vi "Measurement Parser.vi"(8 "error in (no error)":errorcluster, 9 "Universal Power Meter.lvlib:Universal Card.lvclass":refnum<class "Universal Card.lvclass">, 10 "Data Array":dbl[](array[numeric]), 11 "Yokogawa WT500 in":refnum<class "Yokogawa WT500.lvclass">) -> (0 "error out":errorcluster, 2 "Waveform Graph":dynamicdata(graph), 3 "Yokogawa WT500 out":refnum<class "Yokogawa WT500.lvclass">)   [LabVIEW 2013, in "Universal Power Meter.lvlib" / "Yokogawa WT500.lvlib" / "Yokogawa WT500.lvclass"]
uses:
  Yokogawa WT500.lvclass
  Universal Card Class/Universal Card.lvclass
  Measured Value Header Control.ctl
  Universal Card Class/Universal Card.lvclass/Universal Card.ctl
  Generic Instrument/Generic Card/Generic Card.lvclass/Generic Card.ctl
  Generic Instrument/Generic Card/Generic Card.lvclass
  Data Logger/Data Logger.lvclass
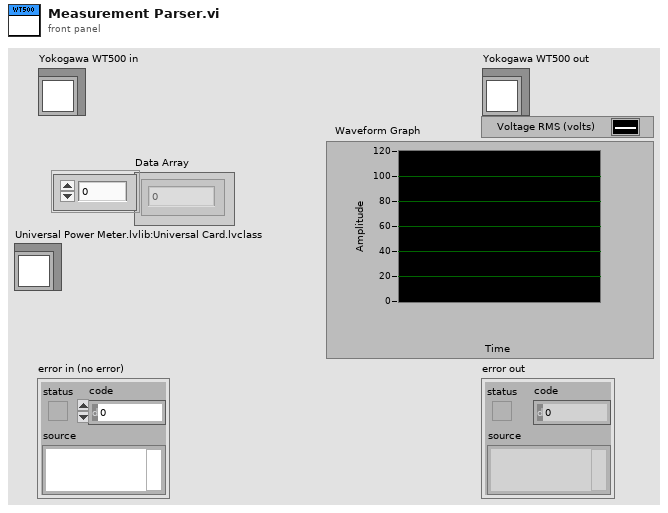
[diagram p1: front panel]
types:
  T1 = typedef "Measured Value Header Control.ctl" = enum16{"Power factor", "Current THD (%)", "Voltage THD (%)", "Amp-Hours", "Energy (Watt-hours)", "Frequency (Herts)", "Power (watts)", "Current RMS (amps)", "Voltage RMS (volts)"}
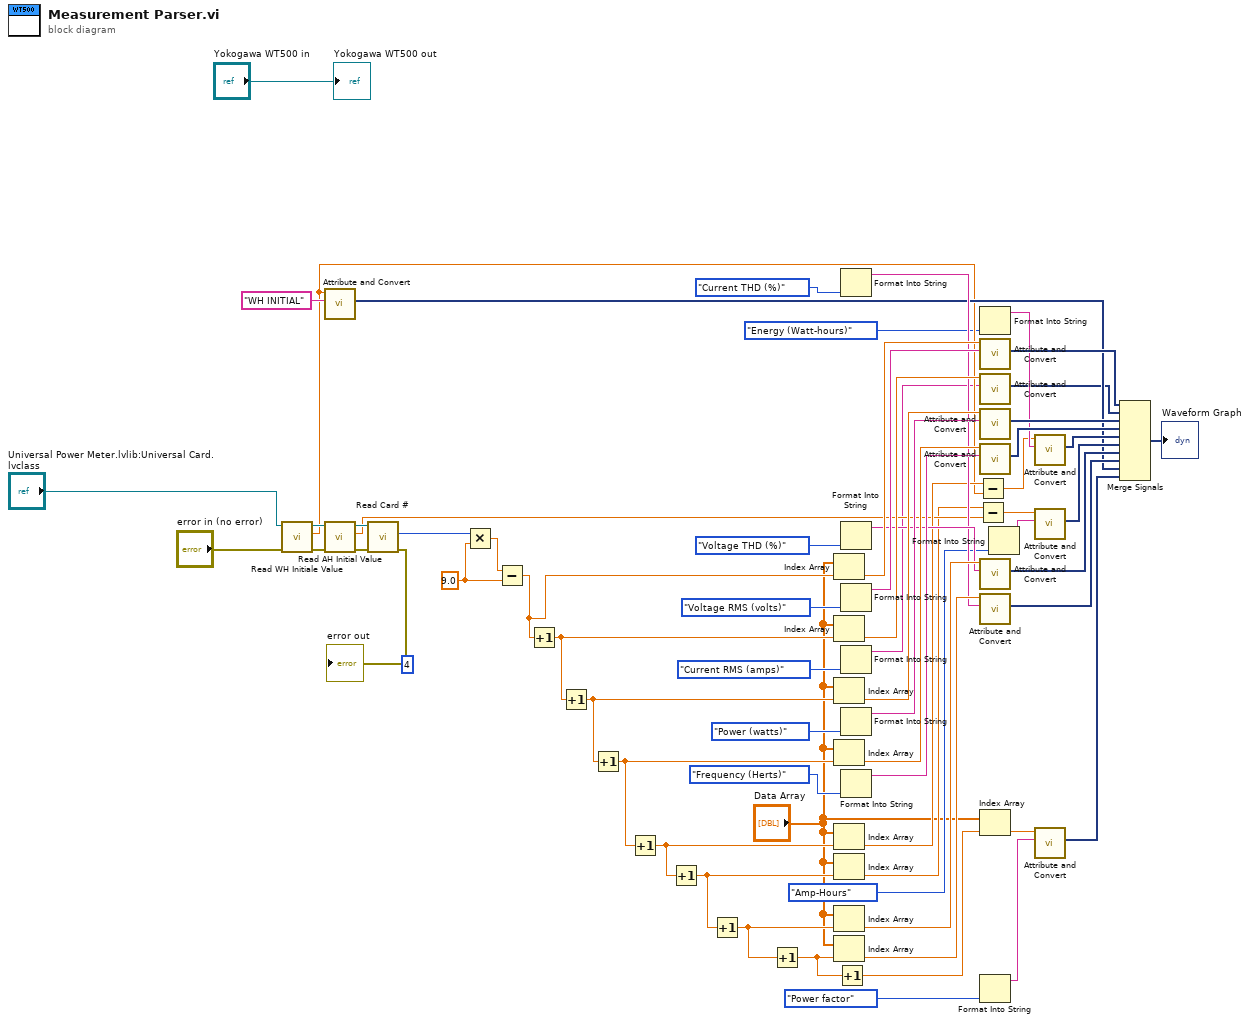
[diagram p0: block diagram]
diagram:
  w3 = 9.0 ("y")
  (unwired) u8 4 ("y")
  n1 = call "Read WH Initiale Value.vi"("error in (no error)"="error in (no error)", "Universal Card in"="Universal Power Meter.lvlib:Universal Card.lvclass") -> ("error out"=w32:errorcluster, "WH Initiale Value"=w20:dbl, "Universal Card out"=w33:refnum<class "Universal Card.lvclass">)  [unwired: 7 in]
  n2 = call "Attribute and Convert.vi"("Signal Name"="WH INITIAL", "Number in"=w20) -> ("Dynamic Signal Out"=w21:dynamicdata)  [unwired: 9 in]
  n3 = call "Read AH Initial Value.vi"("error in (no error)"=w32, "Universal Card in"=w33) -> ("error out"=w30:errorcluster, "AH Initial Value"=w25:dbl, "Universal Card out"=w28:refnum<class "Universal Card.lvclass">)  [unwired: 7 in]
  n4 = call "Read Card #.vi"("error in (no error)"=w30, "Generic Card in"=w28) -> ("error out"=→"error out":errorcluster, "Card #"=w5:u8)  [unwired: 7 in, 1 out]
  n5 = Multiply(x=w5, y=w3) -> (x*y=w4:dbl)
  n6 = Subtract(x=w4, y=w3) -> (x-y=w50:dbl)
  n7 = Increment(x=w50) -> (x+1=w53:dbl)
  n8 = Increment(x=w53) -> (x+1=w55:dbl)
  n9 = Increment(x=w55) -> (x+1=w57:dbl)
  n10 = Increment(x=w57) -> (x+1=w58:dbl)
  n11 = Increment(x=w58) -> (x+1=w45:dbl)
  n12 = Increment(x=w45) -> (x+1=w43:dbl)
  n13 = Increment(x=w43) -> (x+1=w9:dbl)
  n14 = Index Array(array="Data Array", index=w50) -> (element=w51:dbl)
  n15 = Index Array(array="Data Array", index=w53) -> (element=w52:dbl)
  n16 = Index Array(array="Data Array", index=w55) -> (element=w54:dbl)
  n17 = Index Array(array="Data Array", index=w57) -> (element=w56:dbl)
  n18 = Index Array(array="Data Array", index=w58) -> (element=w27:dbl)
  n19 = Index Array(array="Data Array", index=w45) -> (element=w24:dbl)
  n20 = Index Array(array="Data Array", index=w43) -> (element=w49:dbl)
  n21 = Index Array(array="Data Array", index=w9) -> (element=w42:dbl)
  n22 = Increment(x=w9) -> (x+1=w8:dbl)
  n23 = Format Into String(Measured_Value_Header_Control."Current THD (%)" ("Strings")) -> (resulting string=w34:string)  [unwired: 3 in, 1 out]
  n24 = Format Into String(Measured_Value_Header_Control."Voltage THD (%)" ("Strings")) -> (resulting string=w35:string)  [unwired: 3 in, 1 out]
  n25 = Format Into String(Measured_Value_Header_Control."Voltage RMS (volts)" ("Strings")) -> (resulting string=w40:string)  [unwired: 3 in, 1 out]
  n26 = Format Into String(Measured_Value_Header_Control."Current RMS (amps)" ("Strings")) -> (resulting string=w1:string)  [unwired: 3 in, 1 out]
  n27 = Format Into String(Measured_Value_Header_Control."Power (watts)" ("Strings")) -> (resulting string=w39:string)  [unwired: 3 in, 1 out]
  n28 = Format Into String(Measured_Value_Header_Control."Frequency (Herts)" ("Strings")) -> (resulting string=w38:string)  [unwired: 3 in, 1 out]
  n29 = Subtract(x=w27, y=w20) -> (x-y=w26:dbl)
  n30 = Subtract(x=w24, y=w25) -> (x-y=w23:dbl)
  n31 = Format Into String(Measured_Value_Header_Control."Energy (Watt-hours)" ("Strings")) -> (resulting string=w37:string)  [unwired: 3 in, 1 out]
  n32 = call "Attribute and Convert.vi"("Signal Name"=w40, "Number in"=w51) -> ("Dynamic Signal Out"=w59:dynamicdata)  [unwired: 9 in]
  n33 = call "Attribute and Convert.vi"("Signal Name"=w1, "Number in"=w52) -> ("Dynamic Signal Out"=w2:dynamicdata)  [unwired: 9 in]
  n34 = call "Attribute and Convert.vi"("Signal Name"=w39, "Number in"=w54) -> ("Dynamic Signal Out"=w60:dynamicdata)  [unwired: 9 in]
  n35 = call "Attribute and Convert.vi"("Signal Name"=w38, "Number in"=w56) -> ("Dynamic Signal Out"=w61:dynamicdata)  [unwired: 9 in]
  n36 = call "Attribute and Convert.vi"("Signal Name"=w35, "Number in"=w49) -> ("Dynamic Signal Out"=w46:dynamicdata)  [unwired: 9 in]
  n37 = call "Attribute and Convert.vi"("Signal Name"=w34, "Number in"=w42) -> ("Dynamic Signal Out"=w44:dynamicdata)  [unwired: 9 in]
  n38 = Index Array(array="Data Array", index=w8) -> (element=w7:dbl)
  n39 = Format Into String(Measured_Value_Header_Control."Power factor" ("Strings")) -> (resulting string=w11:string)  [unwired: 3 in, 1 out]
  n40 = Format Into String(Measured_Value_Header_Control."Amp-Hours" ("Strings")) -> (resulting string=w36:string)  [unwired: 3 in, 1 out]
  n41 = call "Attribute and Convert.vi"("Signal Name"=w37, "Number in"=w26) -> ("Dynamic Signal Out"=w62:dynamicdata)  [unwired: 9 in]
  n42 = call "Attribute and Convert.vi"("Signal Name"=w36, "Number in"=w23) -> ("Dynamic Signal Out"=w63:dynamicdata)  [unwired: 9 in]
  n43 = call "Attribute and Convert.vi"("Signal Name"=w11, "Number in"=w7) -> ("Dynamic Signal Out"=w6:dynamicdata)  [unwired: 9 in]
  n44 = Merge Signals(w59, w2, w60, w61, w62, w63, w46, w44, w21, w6) -> (→"Waveform Graph":dynamicdata)
  "Yokogawa WT500 out" <- "Yokogawa WT500 in"
